vi "my_stft.vi"(4 "Reset":bool, 6 "FFT normalize":bool=TRUE, 7 "force freq bins to power of 2?":bool=TRUE, 8 "window parameter":dbl=nan, 9 "window info":cluster{"type":T1, "length":i32}={"type"=1, "length"=64} {"type" items=["Rectangle"=0, "Hanning"=1, "Hamming"=2, "Blackman-Harris"=3, "Exact Blackman"=4, "Blackman"=5, "Flat Top"=6, "4 Term B-Harris "=7, "7 Term B-Harris"=8, "Low Sidelobe"=9, "Blackman Nuttall"=11, "Triangle"=30, "Bartlett-Hanning"=31, "Bohman"=32, "Parzen"=33, "Welch"=34, "Kaiser"=60, "Dolph-Chebyshev"=61, "Gaussian"=62]}, 10 "time-freq sampling info":cluster{"time steps":i32, "frequency bins":i32}={"time steps"=-1, "frequency bins"=512}, 11 "X":dbl[](array[numeric])) -> (0 "error out":errorcluster, 3 "STFT {X}":cdb[][](array[numeric]) format="%#_4p")   [LabVIEW 2014]
uses:
  <vilib>/Analysis/4window.llb/windowTd.ctl
  <vilib>/Analysis/2dsp.llb/Real FFT.vi
  <vilib>/Analysis/0measdsp.llb/Scaled Time Domain Window (DBL).vi
  <vilib>/Analysis/NI_AALPro.lvlib
  <vilib>/gmath/NI_Gmath.lvlib
panel:
  out "End data buffer":i32
  out "Num steps":i32
  out "Window len":i32
  out "Time step":i32
  out "Padded size":i32
  # "Debug:"
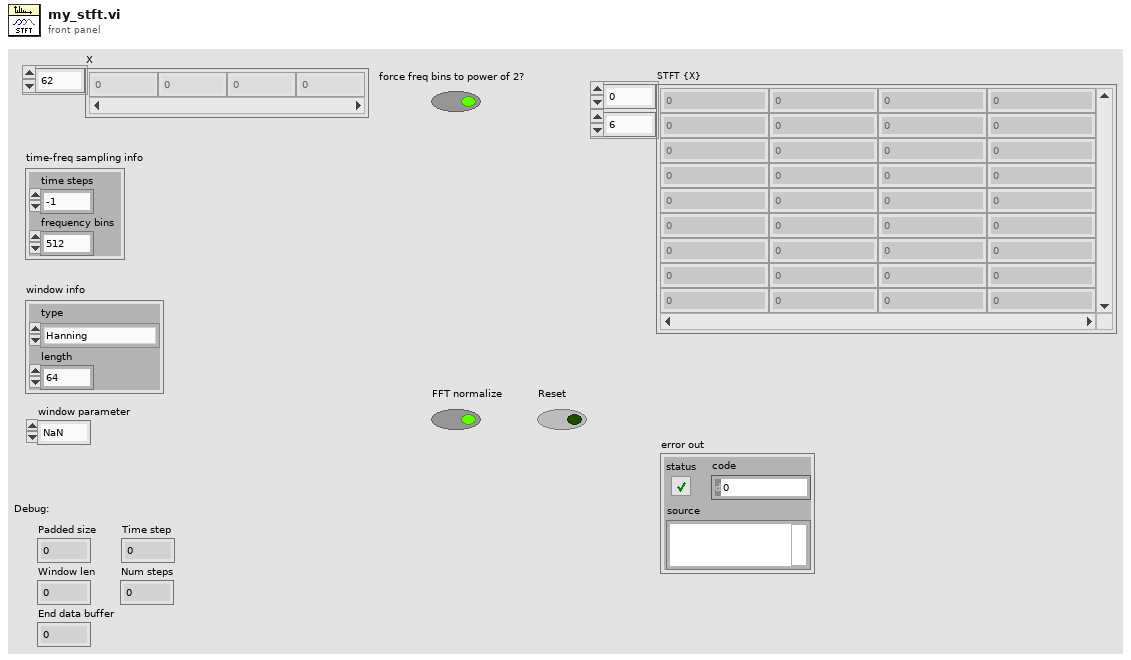
[diagram p1: front panel]
types:
  T1 = typedef "NI_AALPro.lvlib/windowTd.ctl" = u32
  T2 = cluster{"length":i32, "type":T1, "window parameter":dbl}
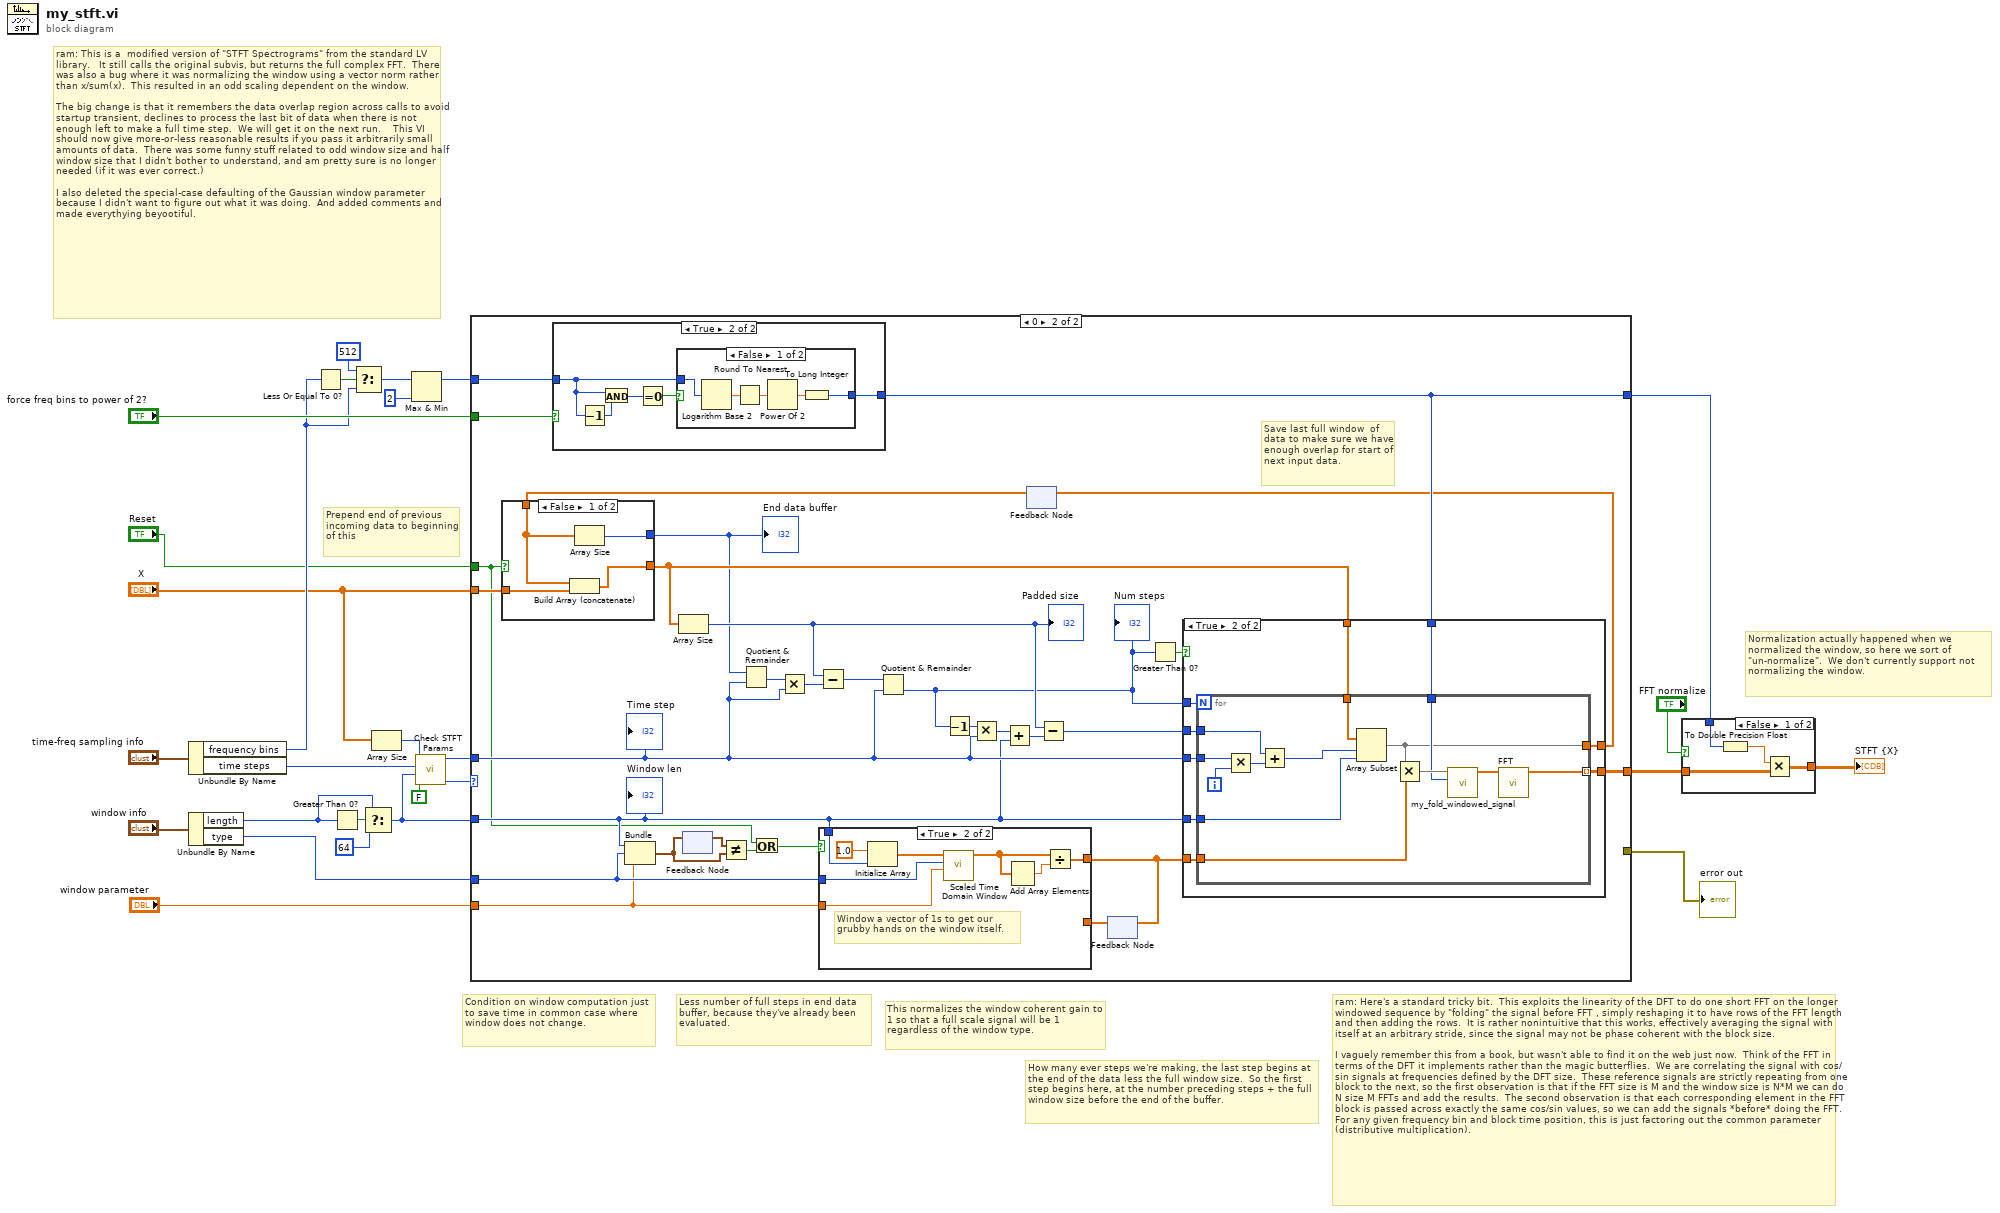
[diagram p0: block diagram]
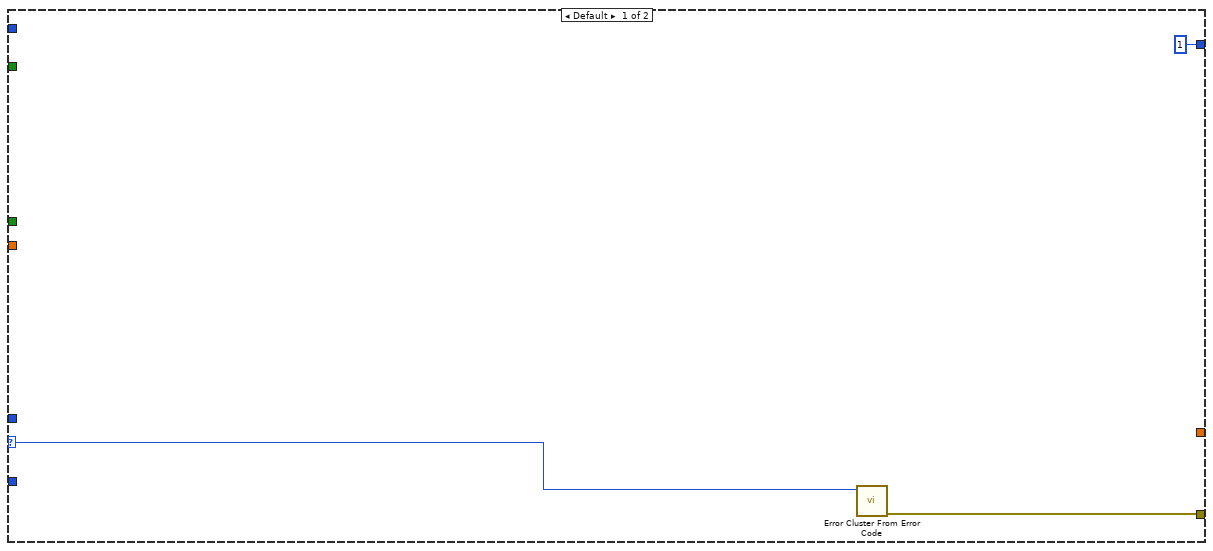
[diagram p3: hidden frame]
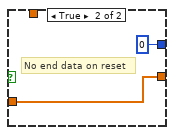
[diagram p4: hidden frame]
diagram:
  # "This normalizes the window coherent gain to 1 so that a full scale signal will be 1 regardless of the window type."
  # "Condition on window computation just to save time in common case where window does not change."
  # "Normalization actually happened when we normalized the window, so here we sort of \"un-normalize\".  We don't currently support not normalizing the window."
  # "How many ever steps we're making, the last step begins at the end of the data less the full window size.  So the first step begins here, at the number preceding steps + the full window size before the end of the buffer."
  # "Less number of full steps in end data buffer, because they've already been evaluated."
  # "Prepend end of previous  incoming data to beginning of this"
  # "ram: Here's a standard tricky bit.  This exploits the linearity of the DFT to do one short FFT on the longer windowed sequence by \"folding\" the signal before FFT , simply reshaping it to have rows of the FFT length and then adding the rows.  It is rather nonintuitive that this works, effectively averaging the signal with itself at an arbitrary stride, since the signal may not be phase coherent with the block size.\n\nI vaguely remember this from a book, but wasn't able to find it on the web just now.  Think of the FFT in terms of the DFT it implements rather than the magic butterflies.  We are correlating the signal with cos/sin signals at frequencies defined by the DFT size.  These reference signals are strictly repeating from one block to the next, so the first observation is that if the FFT size is M and the window size is N*M we can do N size M FFTs and add the results.  The second observation is that each corresponding element in the FFT block is passed across exactly the same cos/sin values, so we can add the signals *before* doing the FFT.  For any given frequency bin and block time position, this is just factoring out the common parameter (distributive multiplication)."
  # "ram: This is a  modified version of \"STFT Spectrograms\" from the standard LV library.   It still calls the original subvis, but returns the full complex FFT.  There was also a bug where it was normalizing the window using a vector norm rather than x/sum(x).  This resulted in an odd scaling dependent on the window.\n\nThe big change is that it remembers the data overlap region across calls to avoid startup transient, declines to process the last bit of data when there is not enough left to make a full time step.  We will get it on the next run.    This VI should now give more-or-less reasonable results if you pass it arbitrarily small amounts of data.  There was some funny stuff related to odd window size and half window size that I didn't bother to understand, and am pretty sure is no longer needed (if it was ever correct.)\n\nI also deleted the special-case defaulting of the Gaussian window parameter because I didn't want to figure out what it was doing.  And added comments and made everythying beyootiful."
  n1 = Unbundle By Name("time-freq sampling info") -> ("frequency bins"=w4:i32, "time steps"=w22:i32)
  n2 = Unbundle By Name("window info") -> ("length"=w20:i32, "type"=w9:T1)
  n3 = Less Or Equal To 0?(x=w4) -> (x <= 0?=w15:bool)
  n4 = Greater Than 0?(x=w20) -> (x > 0?=w25:bool)
  n5 = Select(t=512, s=w15, f=w4) -> (s? t:f=w12:i32)
  n6 = Select(t=w20, s=w25, f=64) -> (s? t:f=w14:i32)
  n7 = Array Size(array="X") -> (size(s)=w27:i32)
  n8 = Max & Min(x=w12, y=2) -> (max(x,y)=w10:i32)  [unwired: 1 out]
  n9 = call <vilib>:"Check STFT Params.vi"("compare signal and window?"=FALSE, "windows length"=w14, "time increment"=w22, "len(X)"=w27) -> ("error"=w26:i32, "time step out"=w19:i32)  [unwired: 6 in]
  n10 = case shown="0" w26 {
    selector: w26 -> [w29 _]
    tunnel: w9 -> [_ w40]
    tunnel: "X" -> [_ w57]
    tunnel: [_ w59] -> w17
    tunnel: w19 -> [_ w44]
    tunnel: "force freq bins to power of 2?" -> [_ w60]
    tunnel: [1 ("frequency bins") w54] -> w16
    tunnel: w14 -> [_ w41]
    tunnel: w10 -> [_ w58]
    tunnel: "window parameter" -> [_ w39]
    tunnel: "Reset" -> [_ w31]
    tunnel: [w28 _] -> w2
    frame Default {
      n11 = call <vilib>:"Error Cluster From Error Code.vi"("error code (0)"=w29) -> ("error out"=w28:errorcluster)  [unwired: 8 in]
    }
    frame 0 {
      # "Save last full window  of data to make sure we have enough overlap for start of next input data."
      n12 = case shown="True" w60 {
        tunnel: w58 -> [w99 w101]
        tunnel: [w99 w100] -> w54
        frame False {
        }
        frame True {
          n13 = Decrement(x=w101) -> (x-1=w104:i32)
          n14 = And(x=w101, y=w104) -> (x .and. y?=w103:i32)
          n15 = Equal To 0?(x=w103) -> (x = 0?=w102:bool)
          n16 = case shown="False" w102 {
            tunnel: w101 -> [w109 w110]
            tunnel: [w105 w110] -> w100
            frame False {
              n17 = Logarithm Base 2(1:w109) -> (0:w108:dbl)
              n18 = Round To Nearest(number=w108) -> (nearest integer value=w107:dbl)
              n19 = Power Of 2(x=w107) -> (2^x=w106:dbl)
              n20 = To Long Integer(number=w106) -> (32bit integer=w105:i32)
            }
            frame True {
            }
          }
        }
      }
      n21 = Bundle("length"=w41, "type"=w40, "window parameter"=w39) -> (w37:T2)  [unwired: 1 in]
      n22 = feedback-in #1(w37) -> ()
      n23 = feedback #1() -> (w38:T2)  [unwired: 1 in]
      n24 = Not Equal?(x=w38, y=w37) -> (x != y?=w36:bool)
      n25 = Or(x=w31, y=w36) -> (x .or. y?=w35:bool)
      n26 = feedback #2() -> (w51:dbl[])  [unwired: 1 in]
      n27 = case shown="False" w31 {
        tunnel: w57 -> [w64 w66]
        tunnel: [w63 w66] -> w55
        tunnel: w51 -> [w62 _]
        tunnel: [w61 0] -> w32
        frame False {
          n28 = Build Array (concatenate)(w62, w64) -> (w63:dbl[])
          n29 = Array Size(array=w62) -> (size(s)=w61:i32)
        }
        frame True {
          # "No end data on reset"
        }
      }
      "End data buffer" <- w32
      n30 = Array Size(array=w55) -> (size(s)=w48:i32)
      "Padded size" <- w48
      n31 = Quotient & Remainder(x=w32, y=w44) -> (floor(x/y)=w50:i32)  [unwired: 1 out]
      n32 = Multiply(x=w50, y=w44) -> (x*y=w49:i32)
      n33 = Subtract(x=w48, y=w49) -> (x-y=w56:i32)
      n34 = Quotient & Remainder(x=w56, y=w44) -> (floor(x/y)=w42:i32)  [unwired: 1 out]
      "Num steps" <- w42
      n35 = Decrement(x=w42) -> (x-1=w43:i32)
      n36 = Multiply(x=w43, y=w44) -> (x*y=w47:i32)
      n37 = Add(x=w47, y=w41) -> (x+y=w46:i32)
      n38 = Subtract(x=w48, y=w46) -> (x-y=w45:i32)
      n39 = feedback #3() -> (w33:dbl[])  [unwired: 1 in]
      n40 = case shown="True" w35 {
        tunnel: [w67 w73] -> w34
        tunnel: w41 -> [_ w70]
        tunnel: w40 -> [_ w69]
        tunnel: w39 -> [_ w68]
        tunnel: w33 -> [w67 _]
        frame False {
          # "Cached window is good"
        }
        frame True {
          # "Window a vector of 1s to get our grubby hands on the window itself."
          n41 = Initialize Array(1.0 ("element"), w70) -> (w74:dbl[])
          n42 = call-poly <vilib>:"Scaled Time Domain Window.vi"("window parameter"=w68, "window"=w69, "X"=w74) -> ("Windowed X"=w72:dbl[])  [unwired: 6 in, 2 out]
          n43 = Add Array Elements(numeric array=w72) -> (sum=w71:dbl)
          n44 = Divide(x=w72, y=w71) -> (x/y=w73:dbl[])
        }
      }
      n45 = feedback-in #3(w34) -> ()
      n46 = Greater Than 0?(x=w42) -> (x > 0?=w53:bool)
      n47 = case shown="True" w53 {
        tunnel: w44 -> [_ w85]
        tunnel: [_ w84] -> w59
        tunnel: w34 -> [_ w83]
        tunnel: w41 -> [_ w82]
        tunnel: w55 -> [w76 w81]
        tunnel: w54 -> [_ w80]
        tunnel: w42 -> [_ w79]
        tunnel: [w76 w78] -> w52
        tunnel: w45 -> [_ w77]
        frame False {
          # "Haven't got a full window of data yet, return empty."
        }
        frame True {
          n48 = for {
            N: w79 -> [_]
            tunnel: w82 -> [w91]
            tunnel: w81 -> [w98]
            tunnel: w85 -> [w94]
            tunnel: w83 -> [w90]
            tunnel: [w92] -> w84 mode=indexing
            tunnel: w80 -> [w93]
            tunnel: [w89] -> w78
            tunnel: w77 -> [w86]
            i -> [w95]
            n49 = Multiply(x=w94, y=w95) -> (x*y=w88:i32)
            n50 = Add(x=w86, y=w88) -> (x+y=w87:i32)
            n51 = Array Subset(array=w98, index=w87, length=w91) -> (w89:dbl[])
            n52 = Multiply(x=w89, y=w90) -> (x*y=w97:dbl[])
            n53 = call "my_fold_windowed_signal.vi"("frequency bins"=w93, "Windowed Signal"=w97) -> ("Folded Signal"=w96:dbl[])  [unwired: 9 in]
            n54 = call-poly <vilib>:"FFT.vi"("X"=w96) -> ("FFT {X}"=w92:cdb[])  [unwired: 9 in, 1 out]
          }
        }
      }
      n55 = feedback-in #2(w52) -> ()
      "Time step" <- w44
      "Window len" <- w41
    }
  }
  "error out" <- w2
  n56 = case shown="False" "FFT normalize" {
    tunnel: w17 -> [w114 w115]
    tunnel: w16 -> [w113 _]
    tunnel: [w112 w115] -> w5
    frame False {
      n57 = To Double Precision Float(number=w113) -> (double precision float=w111:dbl)
      n58 = Multiply(x=w111, y=w114) -> (x*y=w112:cdb[][])
    }
    frame True {
    }
  }
  "STFT {X}" <- w5
